vi "Read Value.vi"(8 "error in (no error)":errorcluster, 11 "int32 in":refnum<class "int32.lvclass">) -> (0 "error out":errorcluster, 2 "Value":i32, 3 "int32 out":refnum<class "int32.lvclass">)   [LabVIEW 2020, in "Protobuf RAW.lvlib" / "int32.lvclass"]
uses:
  int32.lvclass
  int32.lvclass/int32.ctl
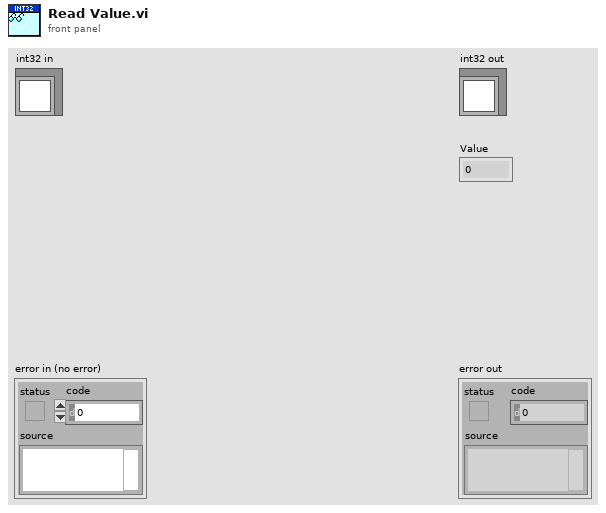
[diagram p1: front panel]
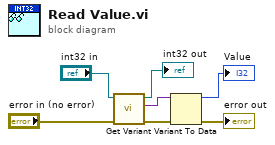
[diagram p0: block diagram]
diagram:
  n1 = call-dynamic "Get Variant.vi"("error in (no error)"="error in (no error)", "Proto Type Common in"="int32 in") -> ("error out"=w2:errorcluster, "Value"=w1:variant, "Proto Type Common out"=→"int32 out":refnum<class "int32.lvclass">)  [unwired: 7 in]
  n2 = Variant To Data(error in=w2, Variant=w1) -> (data=→"Value":i32, error out=→"error out":errorcluster)  [unwired: 1 in]
